vi "2 SailControlFunctionChaos.vi"() -> (2 "Main Sail Position":T1)   [LabVIEW 2011]
uses:
  2 Typedefs/sail setpt.ctl
  0x2-OCU-Think Comm/0x2 Typedefs/Sail Setting Tuning.ctl
  2 Typedefs/apparent wind direction.ctl
  2 Globals/2 Global.vi
  2 Globals/2 TuningConstants.vi
panel:
  out "Jib Position":T1
  out "Sail Setting Options":T2={"Linear\nMode"=FALSE, "Sails Full In Point"=45.0, "Sails Full Out Point"=180.0} {"Sails Full Out Point" step=0.1; "Sails Full In Point" step=0.1}
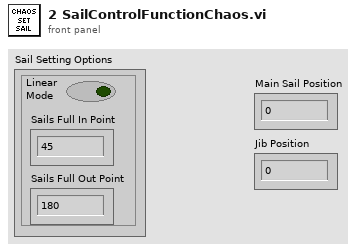
[diagram p1: front panel]
types:
  T1 = typedef "sail setpt.ctl" = dbl
  T2 = typedef "Sail Setting Tuning.ctl" = cluster{"Linear\nMode":bool, "Sails Full In Point":dbl, "Sails Full Out Point":dbl}
  T3 = typedef "apparent wind direction.ctl" = dbl
  T4 = typedef "heading.ctl" = dbl
  T5 = typedef "apparent wind.ctl" = cluster{"Toward Fore":dbl, "Toward Starboard":dbl}
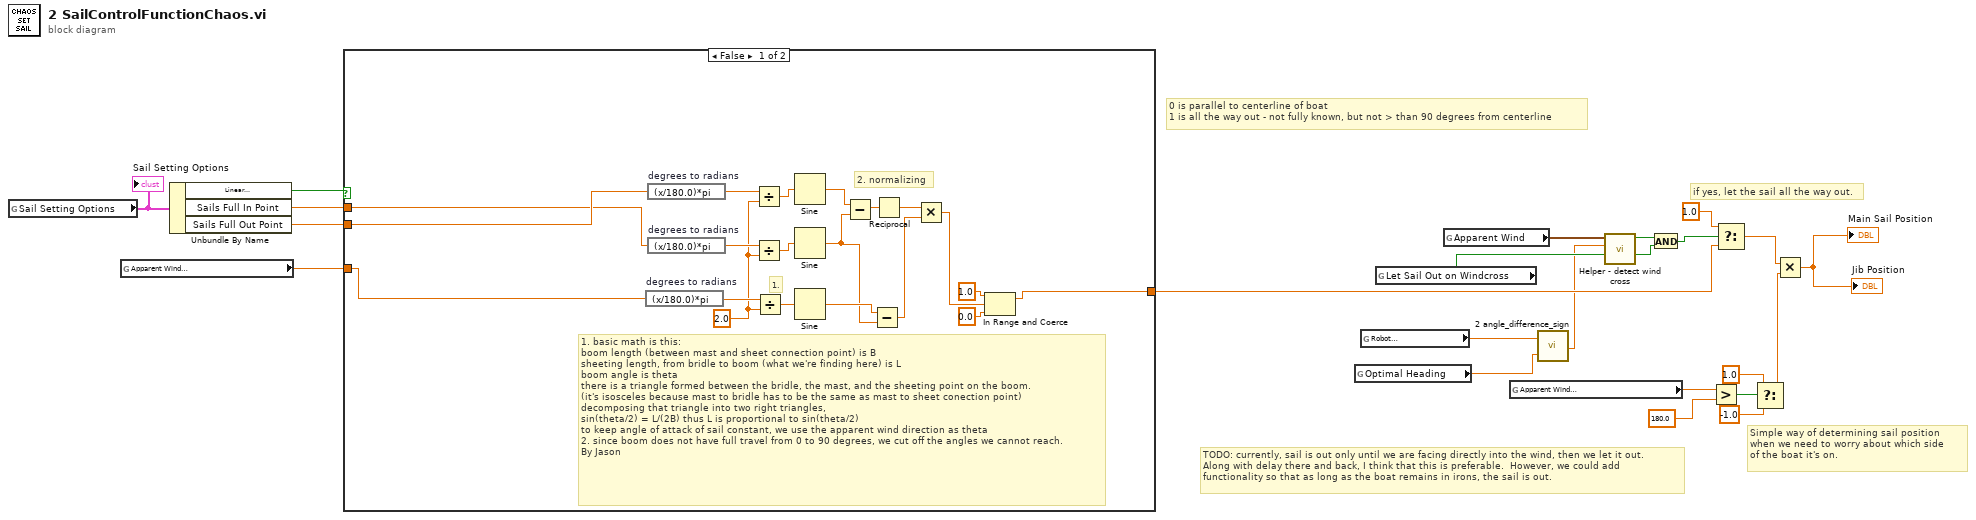
[diagram p0: block diagram]
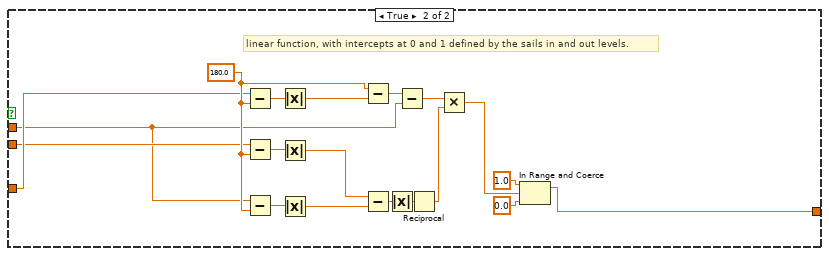
[diagram p2: hidden frame]
diagram:
  # "Simple way of determining sail position\nwhen we need to worry about which side\nof the boat it's on."
  # "TODO: currently, sail is out only until we are facing directly into the wind, then we let it out.\nAlong with delay there and back, I think that this is preferable.  However, we could add \nfunctionality so that as long as the boat remains in irons, the sail is out."
  # "if yes, let the sail all the way out."
  # "0 is parallel to centerline of boat\n1 is all the way out - not fully known, but not > than 90 degrees from centerline"
  n1 = global read "2 TuningConstants.vi" "Sail Setting Options"() -> (w17:T2)
  "Sail Setting Options" <- w17
  n2 = global read "2 Global.vi" "Apparent Wind\nDirection (º)"() -> (w10:T3)
  n3 = Unbundle By Name(w17) -> ("Linear\nMode"=w16:bool, "Sails Full In Point"=w14:dbl, "Sails Full Out Point"=w15:dbl)
  n4 = case shown="False" w16 {
    tunnel: [w27 w45] -> w20
    tunnel: w10 -> [w26 w46]
    tunnel: w15 -> [w25 w44]
    tunnel: w14 -> [w24 w43]
    frame False {
      w28 = 2.0 ("x")
      # "2. normalizing"
      # "1."
      # "1. basic math is this: \nboom length (between mast and sheet connection point) is B\nsheeting length, from bridle to boom (what we're finding here) is L\nboom angle is theta\nthere is a triangle formed between the bridle, the mast, and the sheeting point on the boom.\n(it's isosceles because mast to bridle has to be the same as mast to sheet conection point)\ndecomposing that triangle into two right triangles,\nsin(theta/2) = L/(2B) thus L is proportional to sin(theta/2)\nto keep angle of attack of sail constant, we use the apparent wind direction as theta\n2. since boom does not have full travel from 0 to 90 degrees, we cut off the angles we cannot reach.\nBy Jason"
      n5 = expression code="(x/180.0)*pi" "degrees to radians"(w26) -> (w42:T3)
      n6 = expression code="(x/180.0)*pi" "degrees to radians"(w25) -> (w34:dbl)
      n7 = expression code="(x/180.0)*pi" "degrees to radians"(w24) -> (w37:dbl)
      n8 = Divide(x=w34, y=w28) -> (x/y=w35:dbl)
      n9 = Divide(x=w37, y=w28) -> (x/y=w36:dbl)
      n10 = Divide(x=w42, y=w28) -> (x/y=w41:T3)
      n11 = Sine(x=w35) -> (sin(x)=w33:dbl)
      n12 = Sine(x=w36) -> (sin(x)=w23:dbl)
      n13 = Sine(x=w41) -> (sin(x)=w38:T3)
      n14 = Subtract(x=w33, y=w23) -> (x-y=w32:dbl)
      n15 = Subtract(x=w38, y=w23) -> (x-y=w30:T3)
      n16 = Reciprocal(x=w32) -> (1/x=w31:dbl)
      n17 = Multiply(x=w31, y=w30) -> (x*y=w29:T3)
      n18 = In Range and Coerce(upper limit=1.0, x=w29, lower limit=0.0 ("upper limit")) -> (coerced(x)=w27:T3)  [unwired: 1 out]
    }
    frame True {
      w51 = 180.0 ("upper limit")
      # "linear function, with intercepts at 0 and 1 defined by the sails in and out levels."
      n19 = Subtract(x=w46, y=w51) -> (x-y=w59:T3)
      n20 = Subtract(x=w44, y=w51) -> (x-y=w58:dbl)
      n21 = Subtract(x=w43, y=w51) -> (x-y=w57:dbl)
      n22 = Absolute Value(x=w59) -> (abs(x)=w55:T3)
      n23 = Absolute Value(x=w58) -> (abs(x)=w47:dbl)
      n24 = Absolute Value(x=w57) -> (abs(x)=w48:dbl)
      n25 = Subtract(x=w51, y=w55) -> (x-y=w50:T3)
      n26 = Subtract(x=w47, y=w48) -> (x-y=w56:dbl)
      n27 = Absolute Value(x=w56) -> (abs(x)=w52:dbl)
      n28 = Subtract(x=w50, y=w43) -> (x-y=w49:T3)
      n29 = Reciprocal(x=w52) -> (1/x=w54:dbl)
      n30 = Multiply(x=w49, y=w54) -> (x*y=w53:T3)
      n31 = In Range and Coerce(upper limit=1.0, x=w53, lower limit=0.0 ("upper limit")) -> (coerced(x)=w45:T3)  [unwired: 1 out]
    }
  }
  n32 = global read "2 Global.vi" "Optimal Heading"() -> (w22:dbl)
  n33 = global read "2 Global.vi" "Robot\nHeading"() -> (w9:T4)
  n34 = global read "2 Global.vi" "Let Sail Out on Windcross"() -> (w18:bool)
  n35 = global read "2 Global.vi" "Apparent Wind"() -> (w12:T5)
  n36 = global read "2 Global.vi" "Apparent Wind\nDirection (º)"() -> (w6:T3)
  n37 = call "2 angle_difference_sign.vi"("Angle 2"=w22, "Angle 1"=w9) -> ("Difference"=w11:dbl)
  n38 = call "Helper - detect wind cross.vi"("Heading Change"=w11, "Apparent Wind"=w12) -> ("Crossing Wind?"=w13:bool)  [unwired: 9 in]
  n39 = And(x=w13, y=w18) -> (x .and. y?=w19:bool)
  n40 = Greater?(x=w6, y=T3 180.0) -> (0:w4:bool)
  n41 = Select(t=1.0 ("f"), s=w19, f=w20) -> (s? t:f=w8:T3)
  n42 = Select(t=1.0, s=w4, f=-1.0) -> (s? t:f=w3:dbl)
  n43 = Multiply(x=w8, y=w3) -> (x*y=→"Main Sail Position" →"Jib Position":T3)
